vi "Update State.vi"(8 "error in (no error)":errorcluster, 11 "Simple Sequencer in":refnum<class "Simple Sequencer.lvclass">) -> (0 "error out":errorcluster, 3 "Simple Sequencer out":refnum<class "Simple Sequencer.lvclass">)   [LabVIEW 2018, in "Simple Sequencer.lvclass"]
uses:
  Simple Sequencer.lvclass
  NHMFL_Core/Libraries/Instruments/Sequence/Sequencer State Machine/Sequencer State.ctl
  NHMFL_Core/Libraries/Instruments/Results/Acquired Result/Acquired Result.lvclass
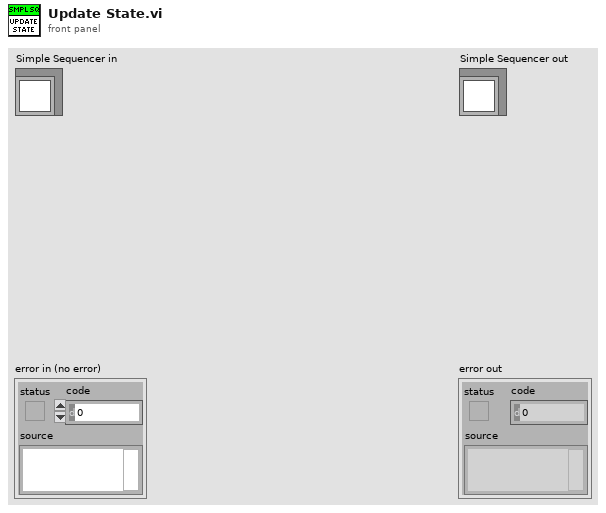
[diagram p1: front panel]
types:
  T1 = typedef "Sequencer State.ctl" = enum16{"Idle", "Starting", "Waiting for primary", "Waiting for secondary"}
  T2 = typedef "Simple Sequencer Configuration.ctl" = cluster{"Primary instrument":string, "Secondary instrument":string, "Start":dbl, "End":dbl, "Step":dbl, "Secondary start":dbl, "Secondary end":dbl}
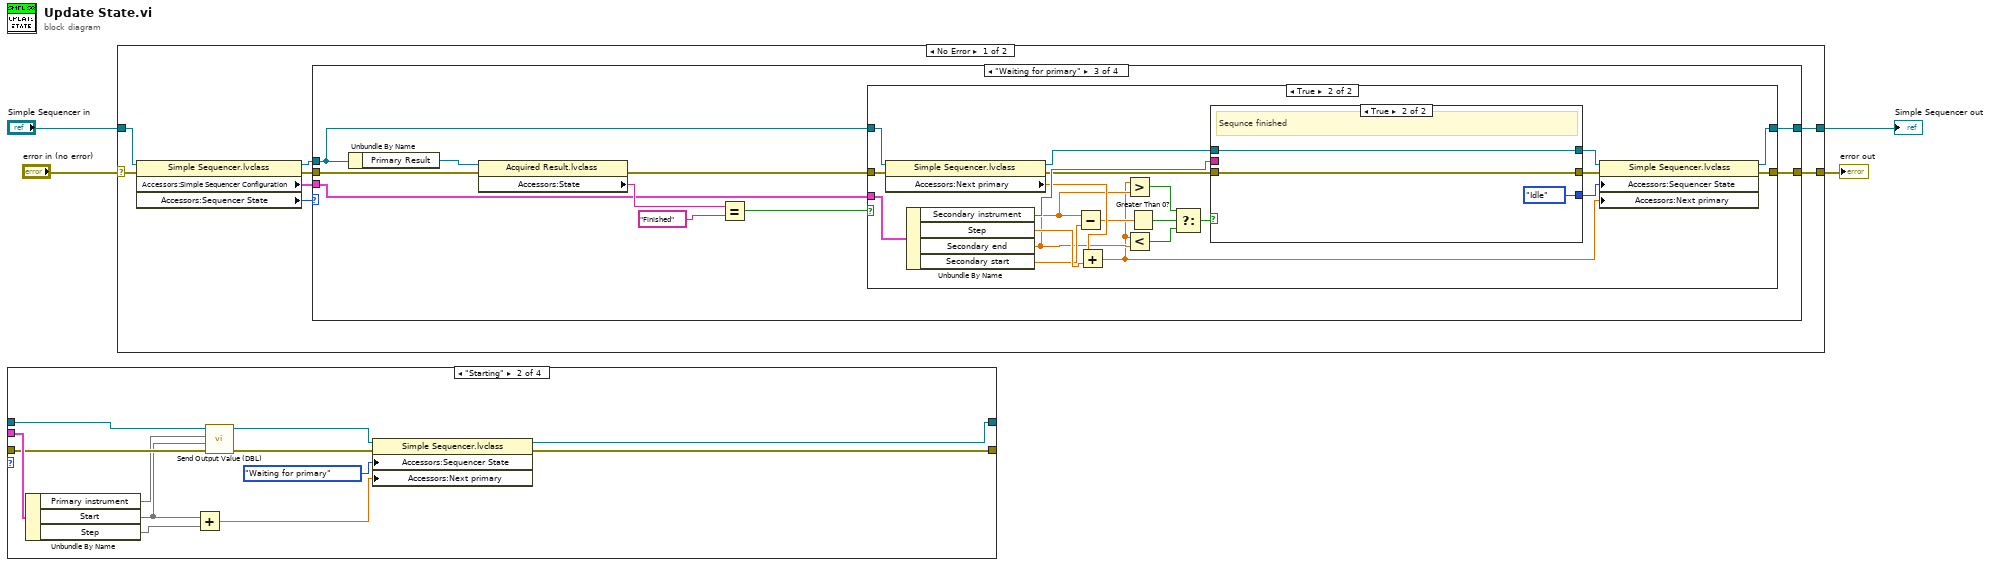
[diagram p0: block diagram]
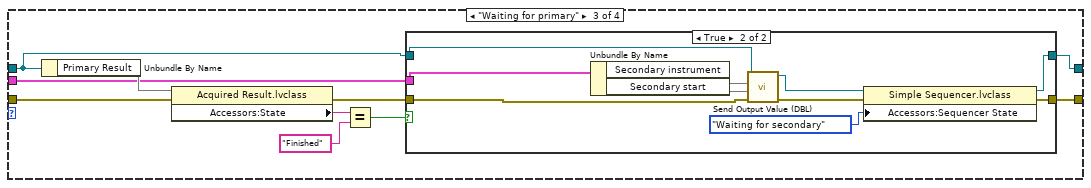
[diagram p3: hidden frame]
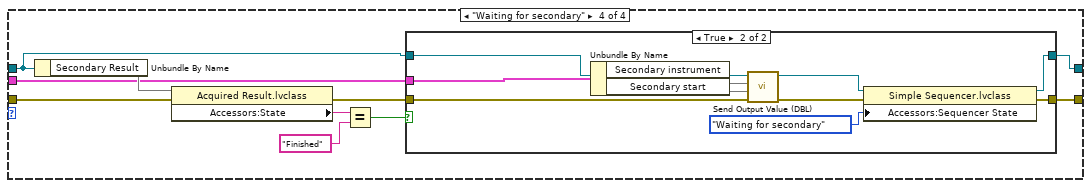
[diagram p5: hidden frame]
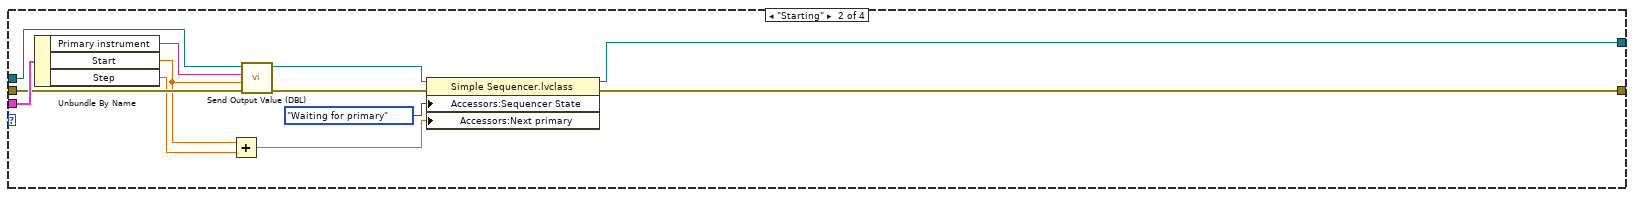
[diagram p8: hidden frame]
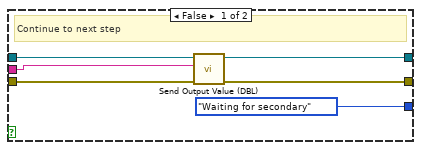
[diagram p10: hidden frame]
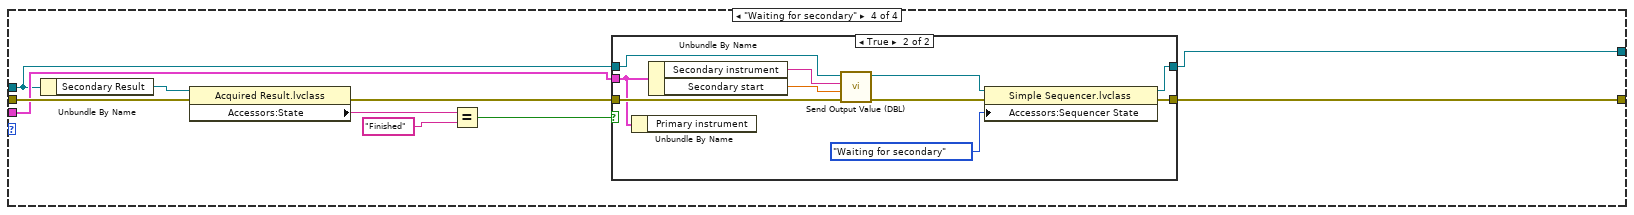
[diagram p11: hidden frame]
diagram:
  n1 = case shown="\"Starting\"" {
    selector: _ -> [_ _ _ _]
    tunnel: _ -> [_ w18 w22 w44]
    tunnel: _ -> [w5 w16 w19 w41]
    tunnel: _ -> [w6 w15 w27 w49]
    tunnel: [w6 w11 w21 w43] -> _
    tunnel: [w5 w10 w20 w42] -> _
    frame "Idle", Default {
    }
    frame "Starting" {
      n2 = Unbundle By Name(w18) -> ("Primary instrument"=w14, "Start"=w9, "Step"=w8)
      n3 = Add(x=w9, y=w8) -> (x+y=w7:dbl)
      n4 = call-dynamic "Send Output Value (DBL).vi"("error in (no error)"=w15, "DBL Value"=w9, "Name"=w14, "Template Module in"=w16) -> ("error out"=w13:errorcluster, "Template Module out"=w12:refnum<class "Simple Sequencer.lvclass">)  [unwired: 6 in]
      n5 = property class="Simple Sequencer.lvclass"(reference=w12, error in=w13, "Accessors:Sequencer State"=Sequencer_State."Waiting for primary" ("Sequencer State"), "Accessors:Next primary"=w7) -> (reference out=w10:refnum<class "Simple Sequencer.lvclass">, error out=w11:errorcluster)
    }
    frame "Waiting for primary" {
      n6 = Unbundle By Name(w19) -> ("Primary Result"=w28)
      n7 = property class="Acquired Result.lvclass"(reference=w28, error in=w27) -> (error out=w23:errorcluster, "Accessors:State"=w26:string)  [unwired: 1 out]
      n8 = Equal?(x=w26, y="Finished") -> (x = y?=w24:bool)
      n9 = case shown="True" w24 {
        tunnel: w22 -> [_ w40]
        tunnel: w19 -> [w29 w38]
        tunnel: w23 -> [w30 w37]
        tunnel: [w30 w33] -> w21
        tunnel: [w29 w32] -> w20
        frame False {
        }
        frame True {
          n10 = Unbundle By Name(w40) -> ("Secondary instrument"=w36, "Secondary start"=w31)
          n11 = call-dynamic "Send Output Value (DBL).vi"("error in (no error)"=w37, "DBL Value"=w31, "Name"=w36, "Template Module in"=w38) -> ("error out"=w35:errorcluster, "Template Module out"=w34:refnum<class "Simple Sequencer.lvclass">)  [unwired: 6 in]
          n12 = property class="Simple Sequencer.lvclass"(reference=w34, error in=w35, "Accessors:Sequencer State"=Sequencer_State."Waiting for secondary" ("Sequencer State")) -> (reference out=w32:refnum<class "Simple Sequencer.lvclass">, error out=w33:errorcluster)
        }
      }
    }
    frame "Waiting for secondary" {
      n13 = Unbundle By Name(w41) -> ("Secondary Result"=w50)
      n14 = property class="Acquired Result.lvclass"(reference=w50, error in=w49) -> (error out=w45:errorcluster, "Accessors:State"=w48:string)  [unwired: 1 out]
      n15 = Equal?(x=w48, y="Finished") -> (x = y?=w46:bool)
      n16 = case shown="True" w46 {
        tunnel: w44 -> [_ w62]
        tunnel: w41 -> [w51 w60]
        tunnel: w45 -> [w52 w59]
        tunnel: [w52 w55] -> w43
        tunnel: [w51 w54] -> w42
        frame False {
        }
        frame True {
          n17 = Unbundle By Name(w62) -> ("Secondary instrument"=w58, "Secondary start"=w53)
          n18 = call-dynamic "Send Output Value (DBL).vi"("error in (no error)"=w59, "DBL Value"=w53, "Name"=w58, "Template Module in"=w60) -> ("error out"=w57:errorcluster, "Template Module out"=w56:refnum<class "Simple Sequencer.lvclass">)  [unwired: 6 in]
          n19 = property class="Simple Sequencer.lvclass"(reference=w56, error in=w57, "Accessors:Sequencer State"=Sequencer_State."Waiting for secondary" ("Sequencer State")) -> (reference out=w54:refnum<class "Simple Sequencer.lvclass">, error out=w55:errorcluster)
        }
      }
    }
  }
  n20 = case shown="No Error" "error in (no error)" {
    selector: "error in (no error)" -> [w70 w150]
    tunnel: [w64 w150] -> w3
    tunnel: [w63 w149] -> w1
    tunnel: "Simple Sequencer in" -> [w69 w149]
    frame No Error {
      n21 = property class="Simple Sequencer.lvclass"(reference=w69, error in=w70) -> (reference out=w66:refnum<class "Simple Sequencer.lvclass">, error out=w65:errorcluster, "Accessors:Simple Sequencer Configuration"=w68:T2, "Accessors:Sequencer State"=w67:T1)
      n22 = case shown="\"Waiting for primary\"" w67 {
        tunnel: w68 -> [_ w84 w88 w130]
        tunnel: w66 -> [w71 w82 w85 w127]
        tunnel: w65 -> [w72 w81 w93 w135]
        tunnel: [w72 w77 w87 w129] -> w64
        tunnel: [w71 w76 w86 w128] -> w63
        frame "Idle", Default {
        }
        frame "Starting" {
          n23 = Unbundle By Name(w84) -> ("Primary instrument"=w80:string, "Start"=w75:dbl, "Step"=w74:dbl)
          n24 = Add(x=w75, y=w74) -> (x+y=w73:dbl)
          n25 = call-dynamic "Send Output Value (DBL).vi"("error in (no error)"=w81, "DBL Value"=w75, "Name"=w80, "Template Module in"=w82) -> ("error out"=w79:errorcluster, "Template Module out"=w78:refnum<class "Simple Sequencer.lvclass">)  [unwired: 6 in]
          n26 = property class="Simple Sequencer.lvclass"(reference=w78, error in=w79, "Accessors:Sequencer State"=Sequencer_State."Waiting for primary" ("Sequencer State"), "Accessors:Next primary"=w73) -> (reference out=w76:refnum<class "Simple Sequencer.lvclass">, error out=w77:errorcluster)
        }
        frame "Waiting for primary" {
          n27 = Unbundle By Name(w85) -> ("Primary Result"=w94:refnum<class "Acquired Result.lvclass">)
          n28 = property class="Acquired Result.lvclass"(reference=w94, error in=w93) -> (error out=w89:errorcluster, "Accessors:State"=w92:string)  [unwired: 1 out]
          n29 = Equal?(x=w92, y="Finished") -> (x = y?=w90:bool)
          n30 = case shown="True" w90 {
            tunnel: w88 -> [_ w117]
            tunnel: w85 -> [w95 w110]
            tunnel: w89 -> [w96 w109]
            tunnel: [w96 w113] -> w87
            tunnel: [w95 w112] -> w86
            frame False {
            }
            frame True {
              n31 = property class="Simple Sequencer.lvclass"(reference=w110, error in=w109) -> (reference out=w111:refnum<class "Simple Sequencer.lvclass">, error out=w108:errorcluster, "Accessors:Next primary"=w107:dbl)
              n32 = Unbundle By Name(w117) -> ("Secondary instrument"=w115:string, "Step"=w106:dbl, "Secondary end"=w102:dbl, "Secondary start"=w105:dbl)
              n33 = Subtract(x=w102, y=w105) -> (x-y=w103:dbl)
              n34 = Add(x=w107, y=w106) -> (x+y=w98:dbl)
              n35 = Greater?(x=w98, y=w102) -> (0:w101:bool)
              n36 = Less?(x=w98, y=w102) -> (x < y?=w100:bool)
              n37 = Greater Than 0?(x=w103) -> (x > 0?=w104:bool)
              n38 = Select(t=w101, s=w104, f=w100) -> (s? t:f=w97:bool)
              n39 = case shown="True" w97 {
                tunnel: [Sequencer_State."Waiting for secondary" ("Sequencer State") Sequencer_State."Idle" ("Sequencer State")] -> w116
                tunnel: w115 -> [w122 _]
                tunnel: [w121 w126] -> w114
                tunnel: w111 -> [w120 w125]
                tunnel: w108 -> [w119 w126]
                tunnel: [w118 w125] -> w99
                frame False {
                  # "Continue to next step"
                  n40 = call-dynamic "Send Output Value (DBL).vi"("error in (no error)"=w119, "Name"=w122, "Template Module in"=w120) -> ("error out"=w121:errorcluster, "Template Module out"=w118:refnum<class "Simple Sequencer.lvclass">)  [unwired: 7 in]
                }
                frame True {
                  # "Sequnce finished"
                }
              }
              n41 = property class="Simple Sequencer.lvclass"(reference=w99, error in=w114, "Accessors:Sequencer State"=w116, "Accessors:Next primary"=w98) -> (reference out=w112:refnum<class "Simple Sequencer.lvclass">, error out=w113:errorcluster)
            }
          }
        }
        frame "Waiting for secondary" {
          n42 = Unbundle By Name(w127) -> ("Secondary Result"=w136:refnum<class "Acquired Result.lvclass">)
          n43 = property class="Acquired Result.lvclass"(reference=w136, error in=w135) -> (error out=w131:errorcluster, "Accessors:State"=w134:string)  [unwired: 1 out]
          n44 = Equal?(x=w134, y="Finished") -> (x = y?=w132:bool)
          n45 = case shown="True" w132 {
            tunnel: w130 -> [_ w139]
            tunnel: w127 -> [w137 w147]
            tunnel: w131 -> [w138 w146]
            tunnel: [w138 w142] -> w129
            tunnel: [w137 w141] -> w128
            frame False {
            }
            frame True {
              n46 = Unbundle By Name(w139) -> ()  [unwired: 1 out]
              n47 = Unbundle By Name(w139) -> ("Secondary instrument"=w145:string, "Secondary start"=w140:dbl)
              n48 = call-dynamic "Send Output Value (DBL).vi"("error in (no error)"=w146, "DBL Value"=w140, "Name"=w145, "Template Module in"=w147) -> ("error out"=w144:errorcluster, "Template Module out"=w143:refnum<class "Simple Sequencer.lvclass">)  [unwired: 6 in]
              n49 = property class="Simple Sequencer.lvclass"(reference=w143, error in=w144, "Accessors:Sequencer State"=Sequencer_State."Waiting for secondary" ("Sequencer State")) -> (reference out=w141:refnum<class "Simple Sequencer.lvclass">, error out=w142:errorcluster)
            }
          }
        }
      }
    }
    frame Error {
    }
  }
  "error out" <- w3
  "Simple Sequencer out" <- w1
